vi "matrix-transpose-benchmark.vi"() -> ()   [LabVIEW 2019]
uses:
  <vilib>/Analysis/Matrix/Datatypes/RealMatrix.ctl
  <vilib>/Analysis/7linalg.llb/Real Transpose Matrix.vi
  <vilib>/Analysis/Matrix/Numeric/Add/Add (Elementwise) - RM,R.vi
  <vilib>/Rock Robotics/WPI/ThirdParty/JAS_Junk/TrajLib/Trajectory_Library.lvlib
  <vilib>/Analysis/NI_AALPro.lvlib
  <vilib>/Analysis/Matrix/NI_Matrix.lvlib
panel:
  out "lin alg add removed":dbl
  out "mtraix add removed":dbl
  out "output matrix":T1
  out "linalg":T1
  out "mat xpose":T1
  out "Add only":dbl format="%18.3f"
  out "LinearAlg Transpose":dbl format="%18.3f"
  out "Matrix transpose":dbl format="%18.3f"
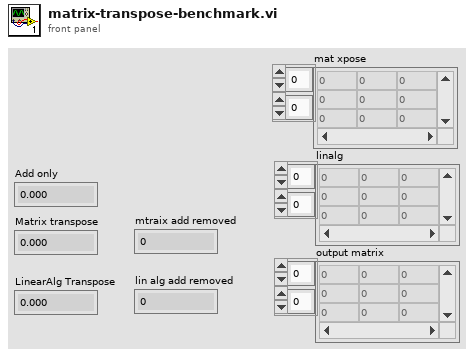
[diagram p1: front panel]
types:
  T1 = typedef "NI_Matrix.lvlib/RealMatrix.ctl" = dbl[][]
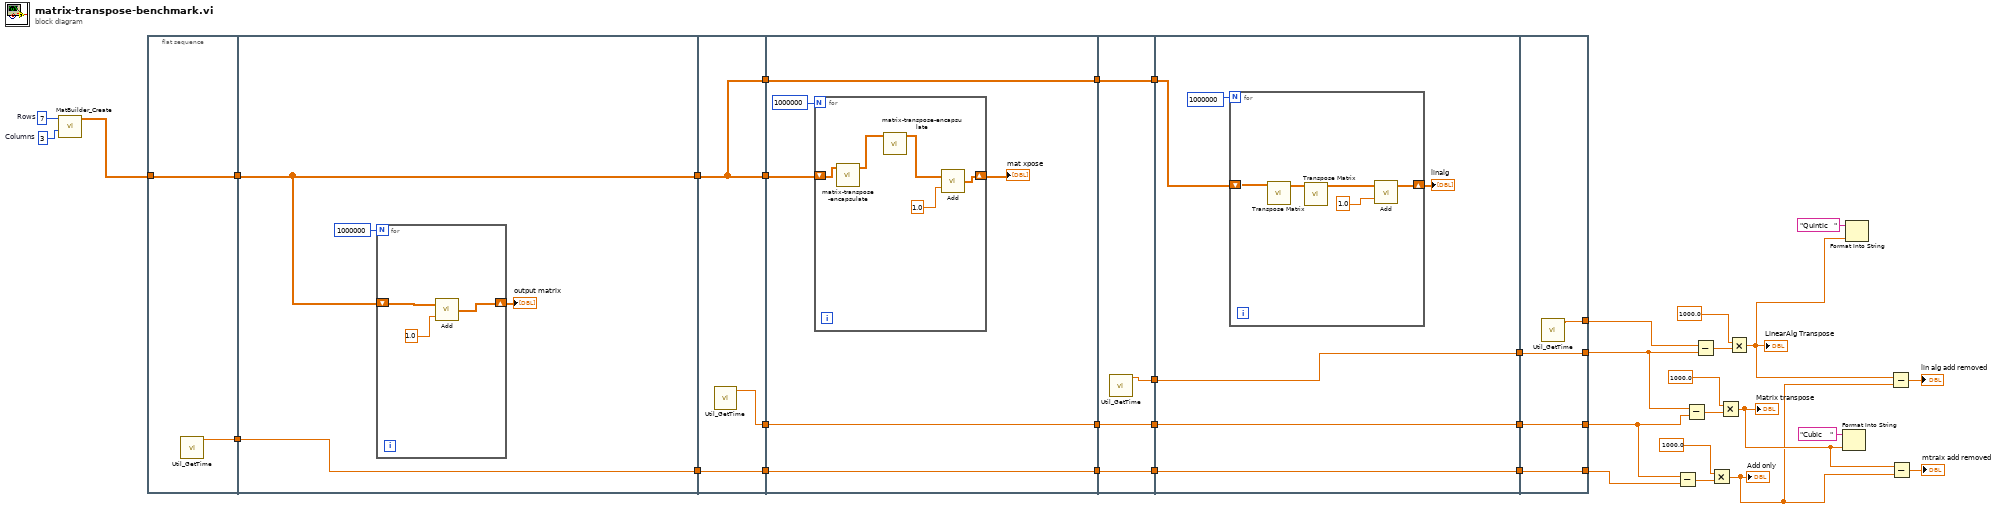
[diagram p0: block diagram]
diagram:
  w25 = 3  # Columns
  w26 = 7  # Rows
  n1 = call <vilib>:"MatBuilder_Create.vi"("Columns"=w25, "Rows"=w26) -> ("output matrix"=w24:T1)  [unwired: 9 in]
  n2 = flat-sequence {
    tunnel: w24 -> [w40]
    tunnel: [w40] -> w18
    tunnel: [w39] -> w10
    tunnel: [w42] -> w19
    tunnel: w18 -> [w42]
    tunnel: [w44] -> w11
    tunnel: w10 -> [w44]
    tunnel: [w50] -> w38
    tunnel: [w49] -> w23
    tunnel: [w49] -> w20
    tunnel: w19 -> [w49]
    tunnel: [w48] -> w12
    tunnel: w11 -> [w48]
    tunnel: w38 -> [w56]
    tunnel: [w56] -> w37
    tunnel: w23 -> [w54]
    tunnel: [w53] -> w21
    tunnel: w20 -> [w53]
    tunnel: [w52] -> w13
    tunnel: w12 -> [w52]
    tunnel: w37 -> [w64]
    tunnel: [w65] -> w34
    tunnel: [w64] -> w29
    tunnel: [w63] -> w22
    tunnel: w21 -> [w63]
    tunnel: [w62] -> w14
    tunnel: w13 -> [w62]
    tunnel: w34 -> [w71]
    tunnel: [w71] -> w31
    tunnel: [w70] -> w30
    tunnel: w29 -> [w70]
    tunnel: w22 -> [w68]
    tunnel: [w67] -> w15
    tunnel: w14 -> [w67]
    tunnel: [w80] -> w17
    tunnel: [w79] -> w16
    tunnel: w31 -> [w79]
    tunnel: [w78] -> w7
    tunnel: w30 -> [w78]
    tunnel: [w77] -> w6
    tunnel: w15 -> [w77]
    frame #0 {
      n3 = call <vilib>:"Util_GetTime.vi"() -> ("FPGA_Time_Seconds"=w39:dbl)  [unwired: 10 in, 1 out]
    }
    frame #1 {
      n4 = for {
        N: 1000000 -> [_]
        shift-right: [w45] -> w41
        shift-left: w42 -> [w46]
        n5 = call-poly <vilib>:"Add.vi"("Real Scalar c"=1.0, "Real Matrix A"=w46) -> ("A + c"=w45:T1)
      }
      "output matrix" <- w41
    }
    frame #2 {
      n6 = call <vilib>:"Util_GetTime.vi"() -> ("FPGA_Time_Seconds"=w50:dbl)  [unwired: 10 in, 1 out]
    }
    frame #3 {
      n7 = for {
        N: 1000000 -> [_]
        shift-right: [w59] -> w51
        shift-left: w54 -> [w61]
        n8 = call "matrix-transpose-encapsulate.vi"("output matrix in"=w61) -> ("output matrix out"=w58:T1)  [unwired: 10 in]
        n9 = call "matrix-transpose-encapsulate.vi"("output matrix in"=w58) -> ("output matrix out"=w57:T1)  [unwired: 10 in]
        n10 = call-poly <vilib>:"Add.vi"("Real Scalar c"=1.0, "Real Matrix A"=w57) -> ("A + c"=w59:T1)
      }
      "mat xpose" <- w51
    }
    frame #4 {
      n11 = call <vilib>:"Util_GetTime.vi"() -> ("FPGA_Time_Seconds"=w65:dbl)  [unwired: 10 in, 1 out]
    }
    frame #5 {
      n12 = for {
        N: 1000000 -> [_]
        shift-right: [w72] -> w66
        shift-left: w68 -> [w76]
        n13 = call-poly <vilib>:"Transpose Matrix.vi"("Input Matrix"=w76) -> ("Matrix Transpose"=w75:T1)  [unwired: 9 in, 1 out]
        n14 = call-poly <vilib>:"Transpose Matrix.vi"("Input Matrix"=w75) -> ("Matrix Transpose"=w73:T1)  [unwired: 9 in, 1 out]
        n15 = call-poly <vilib>:"Add.vi"("Real Scalar c"=1.0, "Real Matrix A"=w73) -> ("A + c"=w72:T1)
      }
      "linalg" <- w66
    }
    frame #6 {
      n16 = call <vilib>:"Util_GetTime.vi"() -> ("FPGA_Time_Seconds"=w80:dbl)  [unwired: 10 in, 1 out]
    }
  }
  n17 = Subtract(x=w7, y=w6) -> (x-y=w9:dbl)
  n18 = Subtract(x=w16, y=w7) -> (x-y=w36:dbl)
  n19 = Subtract(x=w17, y=w16) -> (x-y=w33:dbl)
  n20 = Multiply(x=1000.0, y=w9) -> (x*y=w3:dbl)
  "Add only" <- w3
  n21 = Multiply(x=1000.0, y=w36) -> (x*y=w4:dbl)
  "Matrix transpose" <- w4
  n22 = Multiply(x=1000.0, y=w33) -> (x*y=w5:dbl)
  "LinearAlg Transpose" <- w5
  n23 = Format Into String(initial string="Cubic    ", w4) -> ()  [unwired: 2 in, 2 out]
  n24 = Format Into String(initial string="Quintic   ", w5) -> ()  [unwired: 2 in, 2 out]
  n25 = Subtract(x=w5, y=w3) -> (x-y=→"lin alg add removed":dbl)
  n26 = Subtract(x=w4, y=w3) -> (x-y=→"mtraix add removed":dbl)
